vi "Open Connection.vi"(8 "error in":errorcluster, 10 "password":string, 11 "username":string) -> (0 "error out":errorcluster, 3 "spark reference out":T1)   [LabVIEW 2013, in "Spark API.lvlib"]
doc: "Open a connection to the Spark cloud, and connect to a single online device. If multiple devices are online, this VI will prompt the user to pick one device."
uses:
  Spark API.lvlib
  Controls/Spark Reference.ctl
  <vilib>/httpClient/ClientHandle.ctl
  Controls/Device Query JSON.ctl
  <vilib>/httpClient/LabVIEWHTTPClient.lvlib
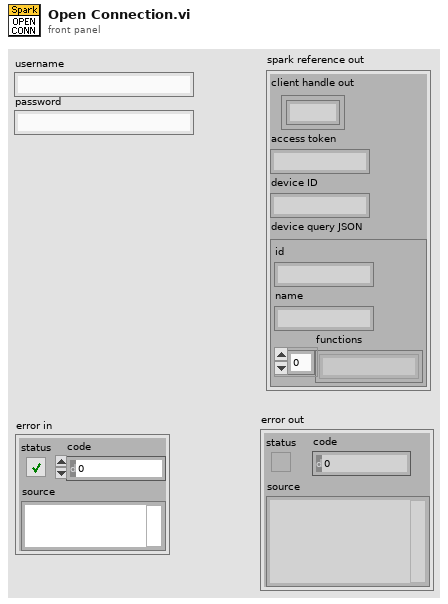
[diagram p1: front panel]
types:
  T1 = typedef "Spark API.lvlib/Spark Reference.ctl" = cluster{"client handle out":T2, "access token":string, "device ID":string, "device query JSON":T3}
  T2 = typedef "LabVIEWHTTPClient.lvlib/ClientHandle.ctl" = refnum<k1>
  T3 = typedef "Spark API.lvlib/Device Query JSON.ctl" = cluster{"id":string, "name":string, "functions":string[]}
  T4 = typedef "Spark API.lvlib/Devices Query JSON.ctl" = cluster{"id":string, "name":string, "connected":bool}[]
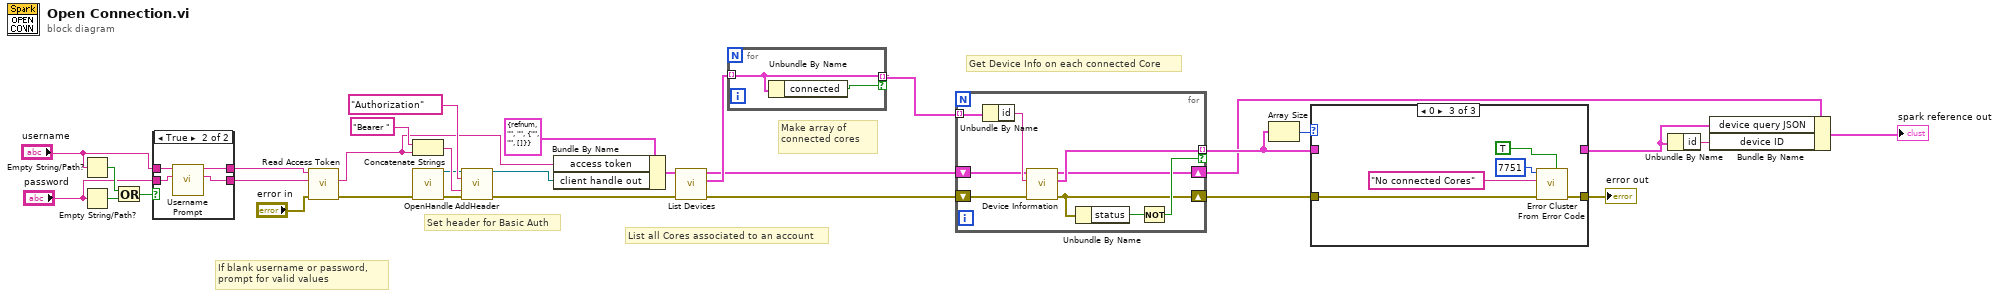
[diagram p0: block diagram]
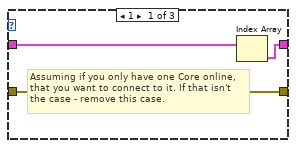
[diagram p3: hidden frame]
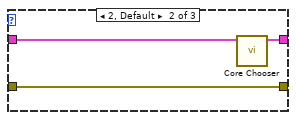
[diagram p4: hidden frame]
diagram:
  # "Get Device Info on each connected Core"
  # "Set header for Basic Auth"
  # "Make array of connected cores"
  # "If blank username or password, prompt for valid values"
  # "List all Cores associated to an account"
  n1 = Empty String/Path?(string/path="username") -> (empty?=w19:bool)
  n2 = Empty String/Path?(string/path="password") -> (empty?=w18:bool)
  n3 = Or(x=w19, y=w18) -> (x .or. y?=w17:bool)
  n4 = case shown="True" w17 {
    tunnel: "username" -> [w33 w37]
    tunnel: "password" -> [w32 w36]
    tunnel: [w33 w35] -> w14
    tunnel: [w32 w34] -> w13
    frame False {
    }
    frame True {
      n5 = call "Username Prompt.vi"("Password"=w36, "Username"=w37) -> ("Password out"=w34:string, "Username out"=w35:string)  [unwired: 8 in]
    }
  }
  n6 = call "Read Access Token.vi"("error in"="error in", "password"=w13, "username"=w14) -> ("error out"=w7:errorcluster, "token"=w3:string)  [unwired: 7 in]
  n7 = Concatenate Strings("Bearer " ("string"), w3) -> (w10:string)
  n8 = call <vilib>:"OpenHandle.vi"("error in (no error)"=w7) -> ("client handle out"=w8:T2, "error out"=w9:errorcluster)  [unwired: 13 in]
  n9 = call <vilib>:"AddHeader.vi"("client handle"=w8, "header"="Authorization", "value"=w10, "error in (no error)"=w9) -> ("client handle out"=w4:T2, "error out"=w6:errorcluster)  [unwired: 10 in]
  n10 = Bundle By Name(cluster=T1 {"client handle out"=refnum, "access token"="", "device ID"="", "device query JSON"={"id"="", "name"="", "functions"=[]}} ("Spark Reference"), "access token"=w3, "client handle out"=w4) -> (w2:T1)
  n11 = call "List Devices.vi"("error in (no error)"=w6, "spark reference in"=w2) -> ("error out"=w20:errorcluster, "devices JSON"=w29:T4, "spark reference out"=w21:T1)  [unwired: 7 in]
  n12 = for {
    tunnel: w29 -> [w39] mode=indexing
    tunnel: [w39] -> w27 mode=indexing if=w38
    n13 = Unbundle By Name(w39) -> ("connected"=w38:bool)
  }
  n14 = for {
    tunnel: w27 -> [w48] mode=indexing
    shift-right: [w42] -> w26
    shift-left: w20 -> [w46]
    tunnel: [w45] -> w25 mode=indexing if=w43
    shift-right: [w41] -> w1
    shift-left: w21 -> [w40]
    n15 = Unbundle By Name(w48) -> ("id"=w47:string)
    n16 = call "Device Information.vi"("error in (no error)"=w46, "id"=w47, "spark reference in"=w40) -> ("error out"=w42:errorcluster, "device query JSON"=w45:T3, "spark reference out"=w41:T1)  [unwired: 6 in]
    n17 = Unbundle By Name(w42) -> ("status"=w44:bool)
    n18 = Not(x=w44) -> (.not. x?=w43:bool)
  }
  n19 = Array Size(array=w25) -> (size(s)=w28:i32)
  n20 = case shown="0" w28 {
    tunnel: w26 -> [w49 w54 w57]
    tunnel: w25 -> [w51 w52 _]
    tunnel: [w50 w53 _] -> w23
    tunnel: [w49 w54 w56] -> w24
    frame 1 {
      # "Assuming if you only have one Core online, that you want to connect to it. If that isn't the case - remove this case."
      n21 = Index Array(array=w51) -> (element=w50:T3)  [unwired: 1 in]
    }
    frame 2, Default {
      n22 = call "Core Chooser.vi"("online cores"=w52) -> ("selected core"=w53:T3)  [unwired: 10 in]
    }
    frame 0 {
      n23 = call <vilib>:"Error Cluster From Error Code.vi"("is warning? (False)"=TRUE ("show call chain? (False)"), "error in (no error)"=w57, "error message (\"\")"="No connected Cores" ("error message (\"\")"), "error code (0)"=7751) -> ("error out"=w56:errorcluster)  [unwired: 5 in]
    }
  }
  "error out" <- w24
  n24 = Unbundle By Name(w23) -> ("id"=w22:string)
  n25 = Bundle By Name(cluster=w1, "device query JSON"=w23, "device ID"=w22) -> (→"spark reference out":T1)
